vi "FC_Get_Target_XML.vi"(7 "Target":T1, 8 "error in":errorcluster) -> (0 "error out":errorcluster, 3 "All Teams XML":string)   [LabVIEW 2013, in "FC_FIRST Client.lvlib"]
doc: "This VI returns the XML data for the given target. The target is either teams or competitions."
uses:
  FC_FIRST Client.lvlib
  FC_Target.ctl
  <vilib>/httpClient/LabVIEWHTTPClient.lvlib
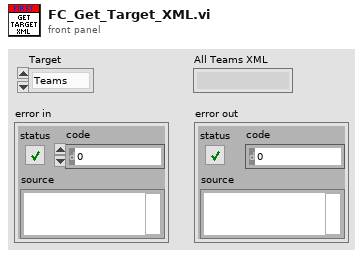
[diagram p1: front panel]
types:
  T1 = typedef "FC_FIRST Client.lvlib/FC_Target.ctl" = enum16{"Teams", "Competitions"}
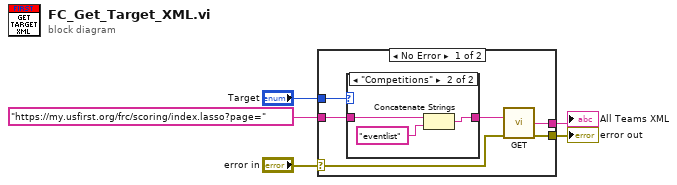
[diagram p0: block diagram]
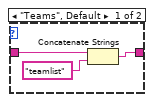
[diagram p2: hidden frame]
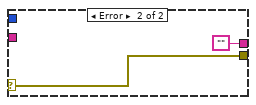
[diagram p3: hidden frame]
diagram:
  n1 = case shown="No Error" "error in" {
    selector: "error in" -> [w6 w19]
    tunnel: [w11 w19] -> w3
    tunnel: "https://my.usfirst.org/frc/scoring/index.lasso?page=" ("URL to List of FIRST Teams") -> [w8 _]
    tunnel: [w10 "" ("body")] -> w2
    tunnel: "Target" -> [w9 _]
    frame No Error {
      n2 = case shown="\"Competitions\"" w9 {
        tunnel: w8 -> [w13 w16]
        tunnel: [w12 w15] -> w7
        frame "Teams", Default {
          n3 = Concatenate Strings(w13, "teamlist" ("URL to List of FIRST Teams")) -> (w12:string)
        }
        frame "Competitions" {
          n4 = Concatenate Strings(w16, "eventlist" ("URL to List of FIRST Teams")) -> (w15:string)
        }
      }
      n5 = call <vilib>:"GET.vi"("url"=w7, "error in (no error)"=w6) -> ("body"=w10:string, "error out"=w11:errorcluster)  [unwired: 10 in, 2 out]
    }
    frame Error {
    }
  }
  "error out" <- w3
  "All Teams XML" <- w2
